vi "dvr_data.vi"(8 "error in (no error)":errorcluster, 11 "dvr":refnum<data-value>) -> (0 "error out":errorcluster, 3 "data":T1={"threads"=[], "MinSize"={"Width"=36, "Height"=36}, "font"={"Font Name"="", "Size"=0, "Bold"=FALSE, "Italic"=FALSE, "Underline"=FALSE, "Strikeout"=FALSE, "Color"=0}})   [LabVIEW 2017, in "rywindow.lvclass"]
uses:
  rywindow.lvclass
  data.ctl
  thread.ctl
  <vilib>/Utility/miscctls.llb/LVFontTypeDef.ctl
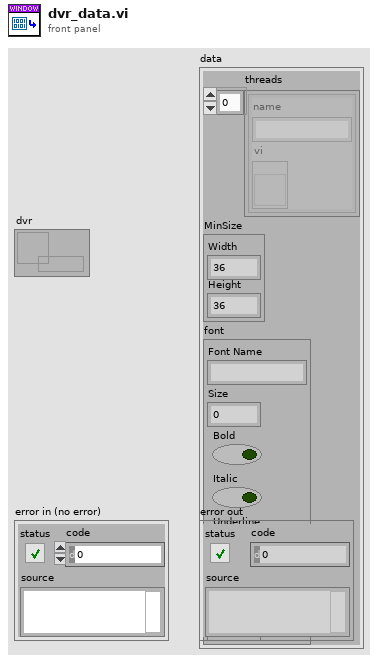
[diagram p1: front panel]
types:
  T1 = typedef "rywindow.lvclass/data.ctl" = cluster{"threads":T2[], "MinSize":cluster{"Width":u32, "Height":u32}, "font":T3}
  T2 = typedef "rywindow.lvclass/thread.ctl" = cluster{"name":string, "vi":refnum<vi>}
  T3 = typedef "LVFontTypeDef.ctl" = cluster{"Font Name":string, "Size":u16, "Bold":bool, "Italic":bool, "Underline":bool, "Strikeout":bool, "Color":u32}
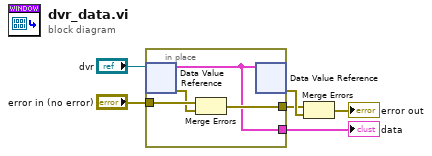
[diagram p0: block diagram]
diagram:
  n1 = in-place {
    in-place-border: "error in (no error)" -> [w10]
    in-place-border: [w8] -> w3
    in-place-border: [w7] -> w6
    n2 = in-place-dvr #1("dvr") -> (w7:T1, w9:errorcluster)
    n3 = Merge Errors(w10, w9) -> (w8:errorcluster)
    n4 = in-place-dvr #1(w7) -> (w4:errorcluster)  [unwired: 1 out]
  }
  "data" <- w6
  n5 = Merge Errors(w3, w4) -> (→"error out":errorcluster)
